vi "delete.vi"(7 "Settings":T1, 8 "error in (no error)":errorcluster, 9 "Args in":string[](array[string]), 10 "String":string, 11 "VISA Refnum in":refnum<visa-resource-name>) -> (0 "error out":errorcluster, 1 "x = y?":bool, 2 "Velocity (units/s)":dbl, 3 "new commands":string, 5 "Args out":string)   [LabVIEW 2020]
uses:
  settings_TypDef.ctl
  shared/numericVariable_TypeDef.ctl
  shared/OnOffTypeDef.ctl
  Direction_TypDef.ctl
  Mode_TypDEf.ctl
  <vilib>/addons/_JKI.lib/Network_Streams_Connection.llb/PublicSettings.ctl
  shared/CompressAndUpdate(Poly)/CompressAndUpdate(Enum).vi
  Newport ESP301/Newport ESP301.lvlib
  BaseDriver/BaseDriver.lvclass
  <vilib>/addons/_JKI.lib/Network_Streams_Connection.llb/NetworkConnection.lvclass
  TapeDrive.lvclass
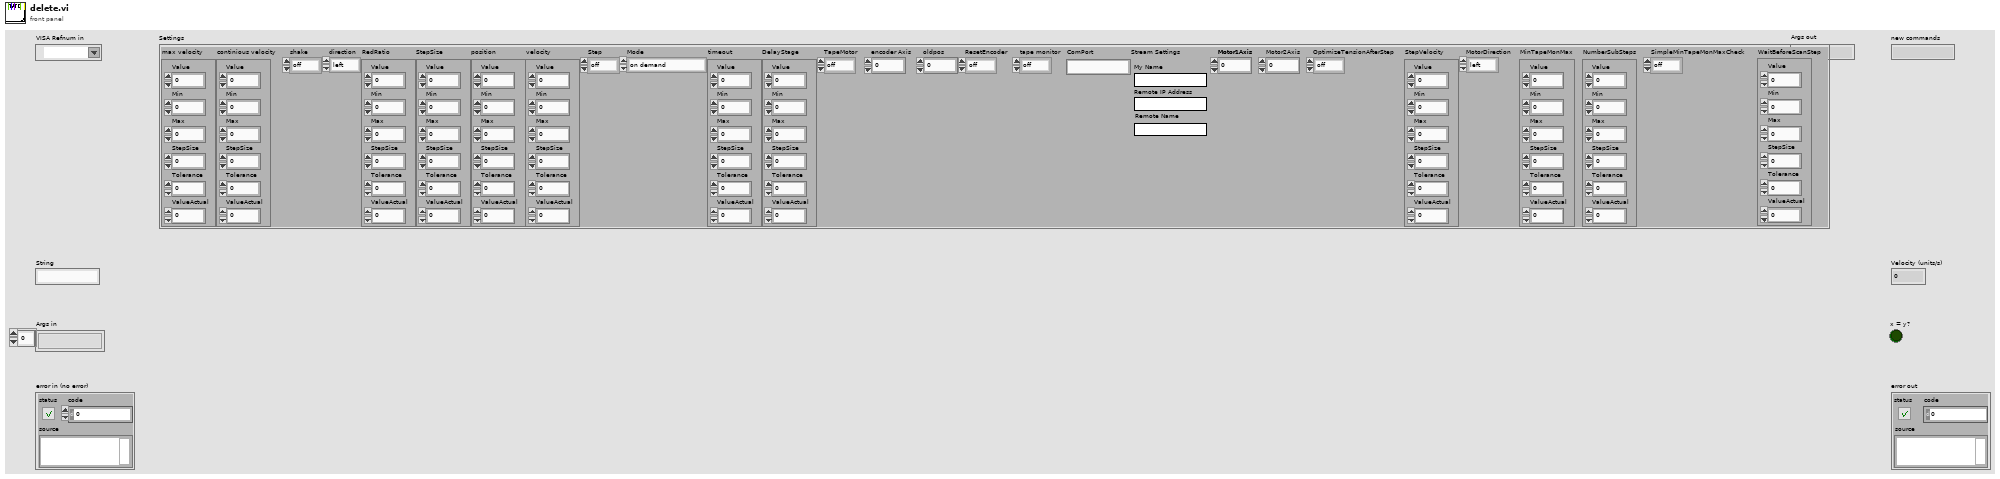
[diagram p1: front panel]
types:
  T1 = typedef "TapeDrive.lvclass/settings_TypDef.ctl" = cluster{"max velocity":T2, "continious velocity":T2, "shake":T3, "direction":T4, "RedRatio":T2, "StepSize":T2, "position":T2, "velocity":T2, "Step":T3, "Mode":T5, "timeout":T2, "DelayStage":T2, "TapeMotor":T3, "encoder Axis":i32, "oldpos":dbl, "ResetEncoder":T3, "tape monitor":T3, "ComPort":string, "Stream Settings":T6, "Motor1Axis":i32, "Motor2Axis":i32, "OptimizeTensionAfterStep":T3, "StepVelocity":T2, "MotorDirection":T4, "MinTapeMonMax":T2, "NumberSubSteps":T2, "SimpleMinTapeMonMaxCheck":T3, "WaitBeforeScanStep":T2}
  T2 = typedef "BaseDriver.lvclass/numericVariable_TypeDef.ctl" = cluster{"Value":dbl, "Min":dbl, "Max":dbl, "StepSize":dbl, "Tolerance":dbl, "ValueActual":dbl}
  T3 = typedef "OnOffTypeDef.ctl" = enum16{"off", "on"}
  T4 = typedef "Direction_TypDef.ctl" = enum16{"left", "right"}
  T5 = typedef "Mode_TypDEf.ctl" = enum16{"on demand", "continuous", "scan"}
  T6 = typedef "NetworkConnection.lvclass/PublicSettings.ctl" = cluster{"My Name":string, "Remote IP Address":string, "Remote Name":string}
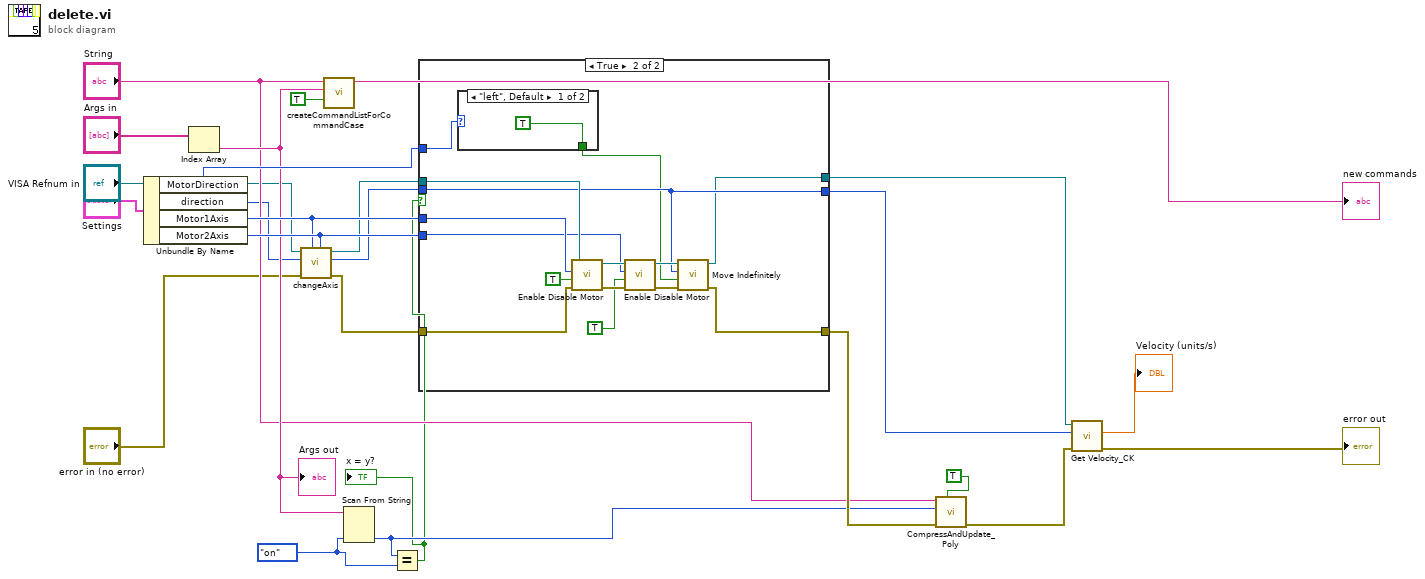
[diagram p0: block diagram]
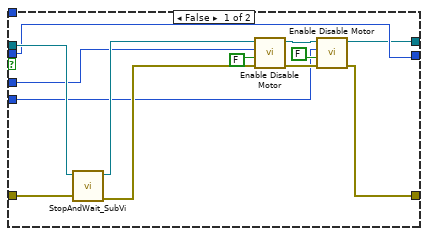
[diagram p2: hidden frame]
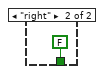
[diagram p3: hidden frame]
diagram:
  w11 = OnOffTypeDef."on" ("TapeMotor")
  n1 = Unbundle By Name("Settings") -> ("MotorDirection"=w25:T4, "direction"=w5:T4, "Motor1Axis"=w23:i32, "Motor2Axis"=w24:i32)
  n2 = Index Array(array="Args in") -> (element=w21:string)  [unwired: 1 in]
  "Args out" <- w21
  n3 = call "changeAxis.vi"("Motor2Axis"=w24, "Motor1Axis"=w23, "error in (no error)"="error in (no error)", "direction 2"=w5, "VISA Refnum in"="VISA Refnum in") -> ("error out"=w9:errorcluster, "Master"=w8:i32, "VISA Refnum out"=w7:refnum<visa-resource-name>)  [unwired: 3 in, 1 out]
  n4 = call "createCommandListForCommandCase.vi"("immediate Check (only once)"=TRUE, "setvalue"=w21, "command"="String") -> ("new commands"=→"new commands":string)  [unwired: 8 in]
  n5 = Scan From String(input string=w21, default 1=w11) -> (output 1=w14:T3)  [unwired: 3 in, 3 out]
  n6 = Equal?(x=w14, y=w11) -> (x = y?=w12:bool)
  "x = y?" <- w12
  n7 = case shown="True" w12 {
    tunnel: w7 -> [w38 w49]
    tunnel: w8 -> [w29 w44]
    tunnel: w9 -> [w37 w47]
    tunnel: [w30 w45] -> w15
    tunnel: [w29 w44] -> w19
    tunnel: [w28 w43] -> w20
    tunnel: w23 -> [w27 w42]
    tunnel: w24 -> [w26 w41]
    tunnel: w25 -> [_ w40]
    frame False {
      n8 = call "StopAndWait_SubVi.vi"("error in (no error)"=w37, "VISA Refnum in"=w38) -> ("error out"=w31:errorcluster, "VISA Refnum out"=w32:refnum<visa-resource-name>)  [unwired: 8 in]
      n9 = call "Enable Disable Motor.vi"("error in (no error)"=w31, "Action (OFF)"=FALSE, "Axis (1)"=w27, "VISA resource name"=w32) -> ("error out"=w34:errorcluster, "VISA resource name out"=w35:refnum<visa-resource-name>)  [unwired: 2 in]
      n10 = call "Enable Disable Motor.vi"("error in (no error)"=w34, "Action (OFF)"=FALSE, "Axis (1)"=w26, "VISA resource name"=w35) -> ("error out"=w30:errorcluster, "VISA resource name out"=w28:refnum<visa-resource-name>)  [unwired: 2 in]
    }
    frame True {
      n11 = case shown="\"left\", Default" w40 {
        tunnel: [TRUE ("Move Direction (+)") FALSE ("Move Direction (+)")] -> w39
        frame "left", Default {
        }
        frame "right" {
        }
      }
      n12 = call "Enable Disable Motor.vi"("error in (no error)"=w47, "Action (OFF)"=TRUE, "Axis (1)"=w42, "VISA resource name"=w49) -> ("error out"=w51:errorcluster, "VISA resource name out"=w52:refnum<visa-resource-name>)  [unwired: 2 in]
      n13 = call "Enable Disable Motor.vi"("error in (no error)"=w51, "Action (OFF)"=TRUE, "Axis (1)"=w41, "VISA resource name"=w52) -> ("error out"=w46:errorcluster, "VISA resource name out"=w48:refnum<visa-resource-name>)  [unwired: 2 in]
      n14 = call "Move Indefinitely.vi"("error in (no error)"=w46, "Move Direction (+)"=w39, "Axis (1)"=w44, "VISA resource name"=w48) -> ("error out"=w45:errorcluster, "VISA resource name out"=w43:refnum<visa-resource-name>)  [unwired: 2 in]
    }
  }
  n15 = call-poly "CompressAndUpdate_Poly.vi"("force CVT update (false)"=TRUE, "error in"=w15, "enum variant"=w14, "command or variable name"="String") -> ("error out"=w18:errorcluster)  [unwired: 7 in]
  n16 = call "Get Velocity_CK.vi"("error in (no error)"=w18, "Axis (1)"=w19, "VISA resource name"=w20) -> ("error out"=→"error out":errorcluster, "Velocity (units/s)"=→"Velocity (units/s)":dbl)  [unwired: 2 in, 1 out]
